vi "Check_if_running.vi"(1 "VI-Pfad":path=path "E:/CryoTUM-Software/16T-Magnet_Ultimate-Control_Version_2-0/LS370Monitor.vi") -> (0 "Running":bool=TRUE)   [LabVIEW 2016]
panel:
  out "LS 370 Monitor":T1(ring)
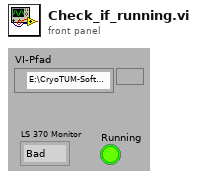
[diagram p1: front panel]
types:
  T1 = enum32{"Bad", "Idle", "Run top level", "Running"}
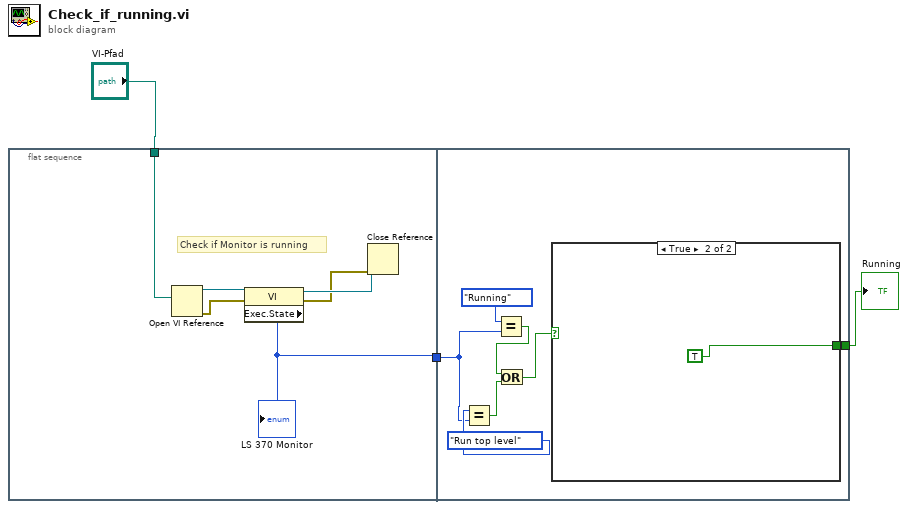
[diagram p0: block diagram]
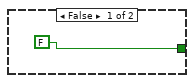
[diagram p2: hidden frame]
diagram:
  n1 = flat-sequence {
    tunnel: [w6] -> w3
    tunnel: "VI-Pfad" -> [w4]
    tunnel: w3 -> [w13]
    tunnel: [w10] -> w1
    frame #0 {
      # "Check if Monitor is running"
      n2 = Open VI Reference(vi path=w4) -> (vi reference=w5:refnum<vi>, error out=w9:errorcluster)  [unwired: 5 in]
      n3 = property class="VI"(reference=w5, error in=w9) -> (reference out=w8:refnum<vi>, error out=w7:errorcluster, "Exec.State"=w6:T1)
      "LS 370 Monitor" <- w6
      n4 = Close Reference(reference=w8, error in (no error)=w7) -> ()  [unwired: 1 out]
    }
    frame #1 {
      n5 = Equal?(x=T1."Run top level" ("LS 370 Monitor 2"), y=w13) -> (x = y?=w12:bool)
      n6 = Equal?(x=T1."Running" ("LS 370 Monitor 2"), y=w13) -> (x = y?=w15:bool)
      n7 = Or(x=w15, y=w12) -> (x .or. y?=w11:bool)
      n8 = case shown="True" w11 {
        tunnel: [FALSE TRUE] -> w10
        frame False {
        }
        frame True {
        }
      }
    }
  }
  "Running" <- w1
